vi "Configure Multicarrier Setup.vi"(0 "VISA resource name":refnum<visa-resource-name>, 1 "Carrier Number (2)":i32=2, 5 "Multicarrier Table Operation (0: Initialize)":u16(ring) items=["Initialize", "Append", "Modify"], 7 "Standard (1: NADC)":u16(ring)=1 items=["GSM"=0, "NADC"=1, "PDC"=2, "PHS"=3, "DECT"=4, "APCO 25 w/C4FM"=5, "APCO w/CQPSK"=6, "CDPD"=7, "PWT"=8, "EDGE"=9, "TETRA"=10, "Select File"=12], 9 "File Name (\"\")":string, 11 "error in (no error)":errorcluster, 12 "Frequency Offset (5 kHz)":dbl=5000.0, 13 "Power (0 dB)":dbl) -> (4 "VISA resource name out":refnum<visa-resource-name>, 15 "error out":errorcluster)   [LabVIEW 2014, in "Agilent PSG MXG Series.lvlib"]
doc: "Configures the carrier type, frequency offset, and power level of the multicarrier table.\n\n<B>Notes:</B>\n(1) This VI is valid only in E8267C, E8267D, N5162A, N5182A, N5172B, N5182B.\n\n(2) For E8267C, this VI is valid only when the instrument installs <B>Option 002</B> (Internal baseband generator) or <B>Option 602</B> (Digital bus baseband generator).\n\n(3) For E8267D, this VI is valid only when the instrument installs <B>Option 601</B> or <B>Option 602</B> (Internal baseband generator).\n\n(4) For N5162A and N5182A, this VI is valid only when the instrument installs <B>Option 651</B> or <B>Option 652</B> or <B>Option 654</B> (Internal baseband generator)."
uses:
  Agilent PSG MXG Series.lvlib
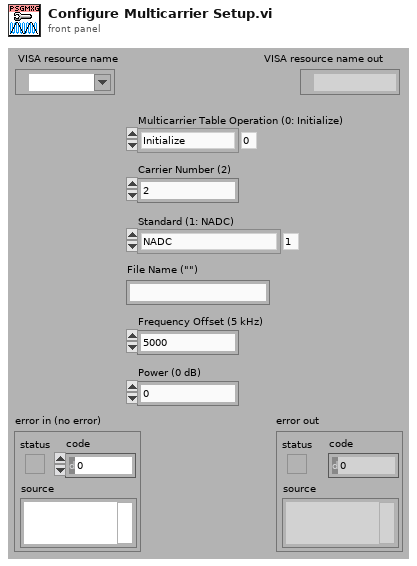
[diagram p1: front panel]
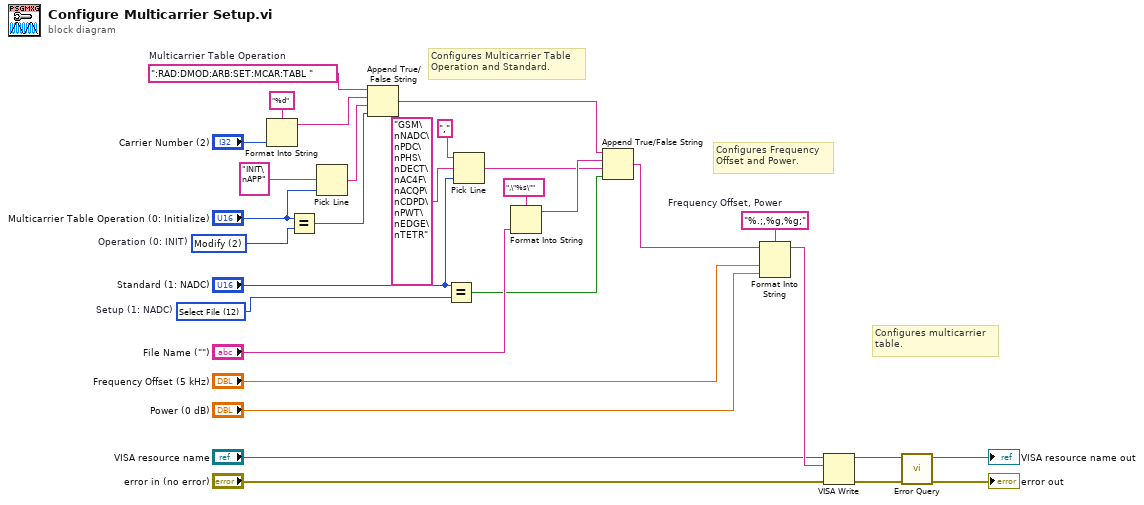
[diagram p0: block diagram]
diagram:
  w5 = u16 12 items=["GSM"=0, "NADC"=1, "PDC"=2, "PHS"=3, "DECT"=4, "APCO 25 w/C4FM"=5, "APCO w/CQPSK"=6, "CDPD"=7, "PWT"=8, "EDGE"=9, "TETRA"=10, "Select File"=12]  # Setup (1: NADC)
  w21 = "%.;,%g,%g;"  # Frequency Offset, Power
  w23 = ":RAD:DMOD:ARB:SET:MCAR:TABL "  # Multicarrier Table Operation
  w30 = u16 2 items=["INIT", "Append", "Modify"]  # Operation (0: INIT)
  # "Configures Frequency\nOffset and Power."
  # "Configures Multicarrier Table\nOperation and Standard."
  # "Configures multicarrier\ntable."
  n1 = Format Into String(format string="%d", "Carrier Number (2)") -> (resulting string=w27:string)  [unwired: 2 in, 1 out]
  n2 = Equal?(x="Multicarrier Table Operation (0: Initialize)", y=w30) -> (x = y?=w24:bool)
  n3 = Pick Line(multi-line string="INIT\nAPP", line index="Multicarrier Table Operation (0: Initialize)") -> (output string=w26:string)  [unwired: 1 out]
  n4 = Append True/False String(1:w24, 2:w26, 3:w27, 4:w23) -> (0:w15:string)
  n5 = Equal?(x="Standard (1: NADC)", y=w5) -> (x = y?=w12:bool)
  n6 = Pick Line(string ("")=",", multi-line string="GSM\nNADC\nPDC\nPHS\nDECT\nAC4F\nACQP\nCDPD\nPWT\nEDGE\nTETR", line index="Standard (1: NADC)") -> (output string=w13:string)
  n7 = Format Into String(format string=",\"%s\"", "File Name (\"\")") -> (resulting string=w14:string)  [unwired: 2 in, 1 out]
  n8 = Append True/False String(1:w12, 2:w13, 3:w14, 4:w15) -> (0:w11:string)
  n9 = Format Into String(format string=w21, initial string=w11, "Frequency Offset (5 kHz)", "Power (0 dB)") -> (resulting string=w8:string)  [unwired: 1 in, 1 out]
  n10 = VISA Write(VISA resource name="VISA resource name", write buffer=w8, error in (no error)="error in (no error)") -> (VISA resource name out=w7:refnum<visa-resource-name>, error out=w6:errorcluster)  [unwired: 1 out]
  n11 = call "Error Query.vi"("error in (no error)"=w6, "VISA resource name"=w7) -> ("error out"=→"error out":errorcluster, "VISA resource name out"=→"VISA resource name out":refnum<visa-resource-name>)  [unwired: 8 out]
